vi "Map Collection - Word Counting.vi"() -> ()   [LabVIEW 2023]
doc: "This VI demonstrates basic use of the map data type. Maps are used to create a collection of keys and associate each unique key with a value. The user selects the two data types used for the keys and for the values.\n\nThis example uses maps to count the occurrences of each word within a block of text."
panel:
  out "Word count as text:":string
  out "Map of word to occurrence count:":map{string, u64}(c390)
  in  "Ignore these words:":string[](array[string])=["the", "an", "a"]
  in  "Count the words in this text:":string="Macbeth by William Shakespeare\nTomorrow, and tomorrow, and tomorrow,\nCreeps in this petty pace from day to day\nTo the last syllable of recorded time,\nAnd all our yesterdays have lighted fools\nThe way to dusty death. Out, out, brief candle!\nLife's but a walking shadow, a poor player\nThat struts and frets his hour upon the stage\nAnd then is heard no more: it is a tale\nTold by an idiot, full of sound and fury,\nSignifying nothing."
  # "Overview: This VI demonstrates basic use of the map data type. Maps are used to create a collection of keys and associate each unique key with a value. The user selects the two data types used for the keys and for the values.\n\nThis example uses maps to count the occurrences of each word within a block of text.\n\nInstructions:\n1. (optional) Change the sample text in the string control. Change the list of ignored words in the array.\n2. Run the VI.  \n3. Observe the output: the map indicator shows all the words that appear in the first string control but not in the array of ignored words. Beside each word is the number of times each word appears in the first string control. This result is displayed both as a map indicator and as a formatted string.\n4. Open the block diagram and review further commentary there."
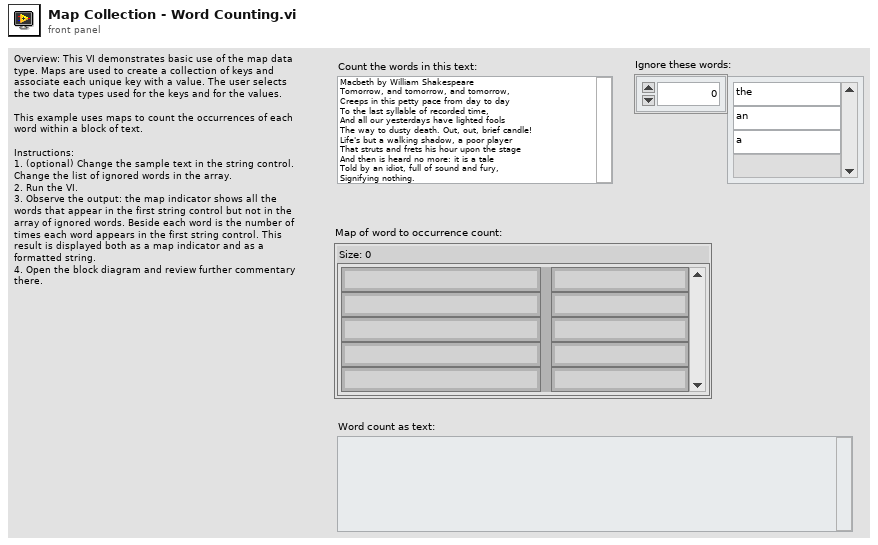
[diagram p1: front panel]
types:
  T1 = enum32{"Modify Entry only if found", "Add or Modify Entry", "Delete Entry"}
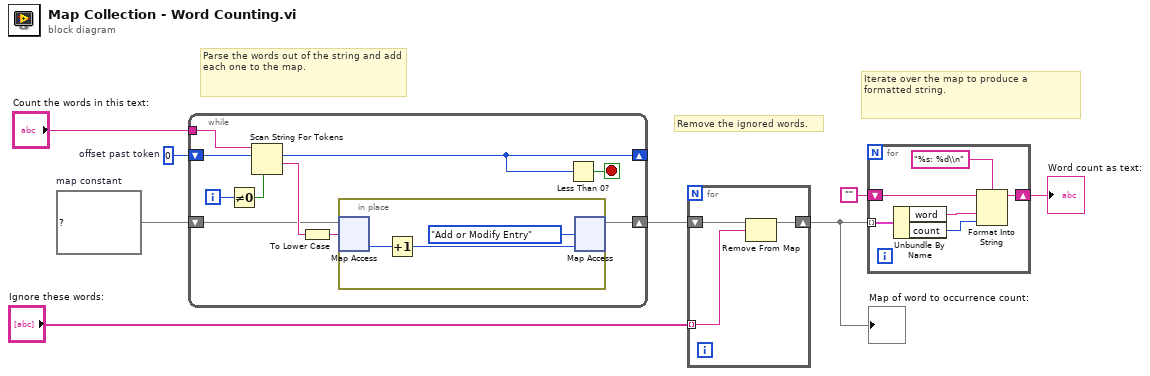
[diagram p0: block diagram]
diagram:
  w6 = map{string, u64} {}  # map constant
  w8 = 0  # offset past token
  # "Parse the words out of the string and add each one to the map."
  # "Iterate over the map to produce a formatted string."
  # "Remove the ignored words."
  n1 = while {
    tunnel: "Count the words in this text:" -> [w17]
    shift-left: w8 -> [w18]
    shift-right: [w9] -> _
    shift-right: [w12] -> w5
    shift-left: w6 -> [w11]
    i -> [w15]
    stop <- w16 stop-if-true
    # "Parse each word."
    n2 = Not Equal To 0?(x=w15) -> (x != 0?=w14:bool)
    n3 = Scan String For Tokens(4:w14, 8:w18, 9:w17) -> (1:w13:string, 2:w9:i32)  [unwired: 3 in, 2 out]
    n4 = To Lower Case(string=w13) -> (all lower case string=w10:string)
    n5 = in-place {
      n6 = in-place-map #1(w11, w10) -> (w21:u64)  [unwired: 1 in, 1 out]
      n7 = Increment(x=w21) -> (x+1=w20:u64)
      n8 = in-place-map #1(w20, T1."Add or Modify Entry" ("action")) -> (w12:map{string, u64})  [unwired: 2 out]
    }
    n9 = Less Than 0?(x=w9) -> (x < 0?=w16:bool)
  }
  n10 = for {
    tunnel: "Ignore these words:" -> [w23] mode=indexing
    shift-right: [w22] -> w3
    shift-left: w5 -> [w24]
    n11 = Remove From Map(10:w23, 11:w24) -> (3:w22:map{string, u64})  [unwired: 2 out]
  }
  "Map of word to occurrence count:" <- w3
  n12 = for {
    tunnel: w3 -> [w30] mode=indexing
    shift-right: [w28] -> w1
    shift-left: "" -> [w27]
    n13 = Unbundle By Name(w30) -> ("word"=w26:string, "count"=w25:u64)
    n14 = Format Into String(format string="%s: %d\\n", initial string=w27, w26, w25) -> (resulting string=w28:string)  [unwired: 1 in, 1 out]
  }
  "Word count as text:" <- w1
